vi "Check Triggers.vi"(7 "Async Data in":T1, 8 "error in (no error)":errorcluster, 10 "Data in":dbl[](array[numeric]), 11 "Waveform Receive in":refnum<class "Waveform Receive.lvclass">) -> (0 "error out":errorcluster, 2 "Data out":dbl[](array[numeric]), 3 "Waveform Receive out":refnum<class "Waveform Receive.lvclass">)   [LabVIEW 2015, in "Waveform Data Logger Engine.lvlib" / "Waveform Receive.lvclass"]
uses:
  Waveform Receive.lvclass
  Types/Async Data.ctl
  <vilib>/NI VeriStand/Custom Device Waveform API/Multiple Waveforms Read (DBL)/Multiple Waveforms Read (DBL).lvclass
  Utilities/Reference Dictionary/Reference Dictionary.lvclass
  Types/Wfm Acq Data.ctl
  Waveform Log/Waveform Log.lvclass
  Types/Async Communication.ctl
  Types/Check File Loop Cmd.ctl
  Waveform Data Logger Engine.lvlib
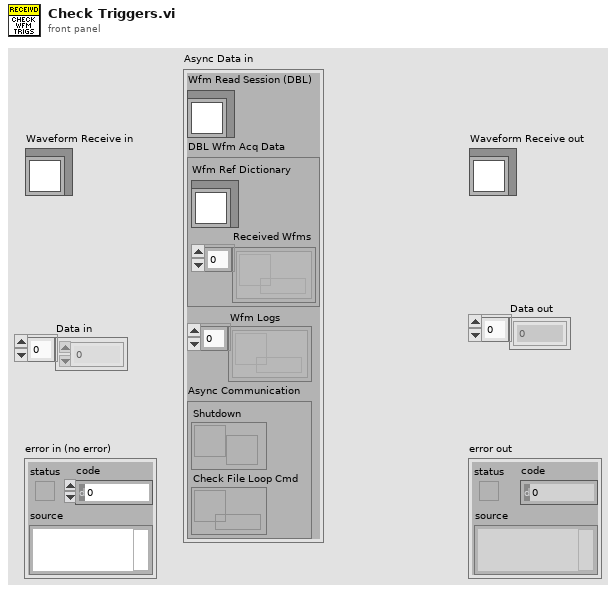
[diagram p1: front panel]
types:
  T1 = typedef "Waveform Data Logger Engine.lvlib/Async Data.ctl" = cluster{"Wfm Read Session (DBL)":refnum<class "Multiple Waveforms Read (DBL).lvclass">, "DBL Wfm Acq Data":T2, "Wfm Logs":refnum<data-value>[], "Async Communication":T3}
  T2 = typedef "Waveform Data Logger Engine.lvlib/Wfm Acq Data.ctl" = cluster{"Wfm Ref Dictionary":refnum<class "Reference Dictionary.lvclass">, "Received Wfms":refnum<data-value>[]}
  T3 = typedef "Waveform Data Logger Engine.lvlib/Async Communication.ctl" = cluster{"Shutdown":refnum<user-event>, "Check File Loop Cmd":refnum<queue>}
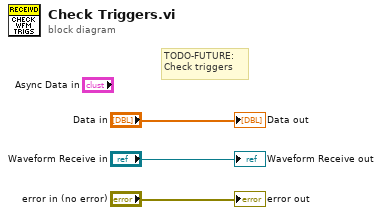
[diagram p0: block diagram]
diagram:
  # "TODO-FUTURE:\nCheck triggers"
  "error out" <- "error in (no error)"
  "Waveform Receive out" <- "Waveform Receive in"
  "Data out" <- "Data in"
